vi "test2.vi"() -> ()   [LabVIEW 2021]
uses:
  IFurniture/IFurniture.lvclass
panel:
  out "error out":errorcluster
  out "price":dbl
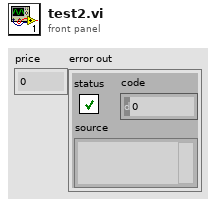
[diagram p1: front panel]
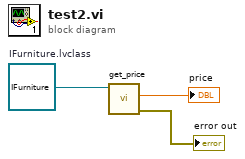
[diagram p0: block diagram]
diagram:
  w3 = refnum<class "IFurniture.lvclass"> refnum  # IFurniture.lvclass
  n1 = call-dynamic "get_price.vi"("IFurniture in"=w3) -> ("error out"=→"error out":errorcluster, "price"=→"price":dbl)  [unwired: 8 in, 1 out]
